vi "Demo how to use.vi"() -> ()   [LabVIEW 2015]
uses:
  <vilib>/Analysis/NI_AALPro.lvlib
panel:
  out "Analog Out":T1
  in  "stop":bool
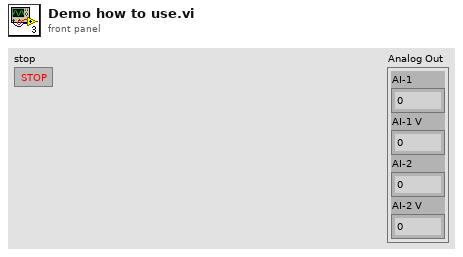
[diagram p1: front panel]
types:
  T1 = cluster{"AI-1":dbl, "AI-1 V":dbl, "AI-2":dbl, "AI-2 V":dbl}
  T2 = cluster{"XInput":dbl[], "Y New Value":dbl[], "Avg point":i16}[]
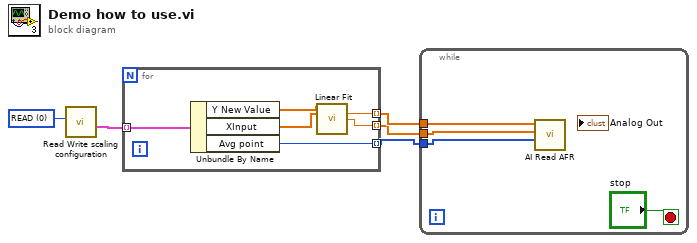
[diagram p0: block diagram]
diagram:
  w5 = u16 0 items=["READ", "WRITE"] ("Read/Write")
  n1 = call "Read Write scaling configuration.vi"("Read/Write"=w5) -> ("Output"=w1:T2)  [unwired: 4 in, 2 out]
  n2 = for {
    tunnel: w1 -> [w11] mode=indexing
    tunnel: [w8] -> w2 mode=indexing
    tunnel: [w7] -> w4 mode=indexing
    tunnel: [w6] -> w3 mode=indexing
    n3 = Unbundle By Name(w11) -> ("Y New Value"=w10:dbl[], "XInput"=w9:dbl[], "Avg point"=w8:i16)
    n4 = call <vilib>:"Linear Fit.vi"("Y"=w10, "X"=w9) -> ("slope"=w7:dbl, "intercept"=w6:dbl)  [unwired: 9 in, 3 out]
  }
  n5 = while {
    tunnel: w4 -> [w14]
    tunnel: w3 -> [w13]
    tunnel: w2 -> [w12]
    stop <- "stop" stop-if-true
    n6 = call "AI Read AFR.vi"("Avg Point"=w12, "Intercept"=w13, "Slope"=w14) -> ()  [unwired: 8 in, 1 out]
  }
